vi "write spi file type2.vi"(8 "milliseconds to wait":u32, 11 "addr/data":string[][](array[string])) -> (3 "res":bool)   [LabVIEW 2018]
uses:
  Dll1_x64_191014_0/Dll1_x64_191014_0.lvlib
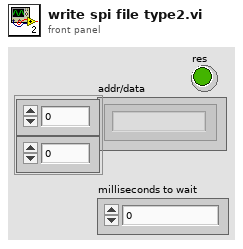
[diagram p1: front panel]
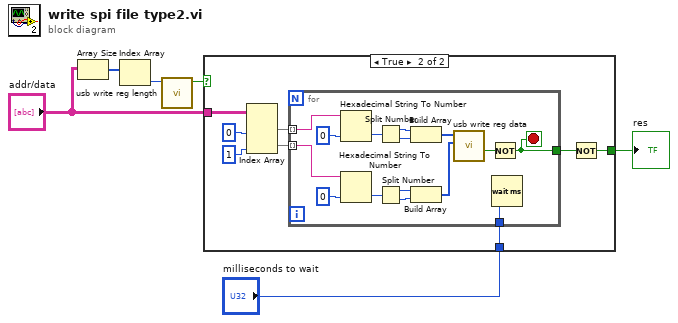
[diagram p0: block diagram]
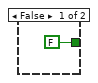
[diagram p2: hidden frame]
diagram:
  n1 = Array Size(array="addr/data") -> (size(s)=w6:i32[])
  n2 = Index Array(array=w6) -> (element=w5:i32)  [unwired: 1 in]
  n3 = call "usb write reg length.vi"("lengthToWrite"=w5) -> ("function return"=w4:bool)  [unwired: 10 in]
  n4 = case shown="True" w4 {
    tunnel: "addr/data" -> [_ w11]
    tunnel: [FALSE w9] -> w2
    tunnel: "milliseconds to wait" -> [_ w8]
    frame False {
    }
    frame True {
      n5 = Index Array(array=w11, index (col) #1=0 ("disabled index (col)"), index (col) #2=1 ("index (col)")) -> (element #1=w14:string[], element #2=w15:string[])  [unwired: 2 in]
      n6 = for {
        tunnel: w14 -> [w28] mode=indexing
        tunnel: w15 -> [w27] mode=indexing
        tunnel: [w17] -> w10
        tunnel: w8 -> [w16]
        stop <- w17 stop-if-true
        n7 = Hexadecimal String To Number(string=w28, default (0uL)=u16 0 ("default (0 U32)")) -> (number=w26:u16)  [unwired: 1 in, 1 out]
        n8 = Hexadecimal String To Number(string=w27, default (0uL)=u16 0 ("default (0 U32)")) -> (number=w25:u16)  [unwired: 1 in, 1 out]
        n9 = Split Number(x=w26) -> (hi(x)=w24:u8, lo(x)=w23:u8)
        n10 = Split Number(x=w25) -> (hi(x)=w22:u8, lo(x)=w21:u8)
        n11 = Build Array(w24, w23) -> (w20:u8[])
        n12 = Build Array(w22, w21) -> (w19:u8[])
        n13 = call "usb write reg data.vi"("write_data"=w19, "addr"=w20) -> ("function return"=w18:bool)  [unwired: 7 in, 2 out]
        n14 = Not(x=w18) -> (.not. x?=w17:bool)
        n15 = Wait (ms)(milliseconds to wait=w16) -> ()  [unwired: 1 out]
      }
      n16 = Not(x=w10) -> (.not. x?=w9:bool)
    }
  }
  "res" <- w2
